vi "UserVars-Plot PDF.vi"(0 "X":dbl[](array[numeric]), 1 "XYGraph":refnum<vi>, 2 "X-axis":refnum<vi>, 5 "PDF":dbl[](array[numeric]), 7 "refpts":dbl[](array[numeric]), 9 "mass":bool, 11 "bernoulli":bool) -> ()   [LabVIEW 2020]
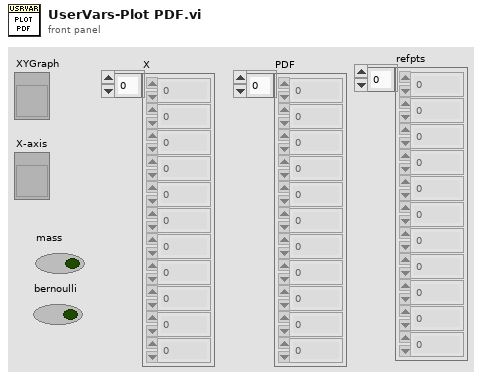
[diagram p1: front panel]
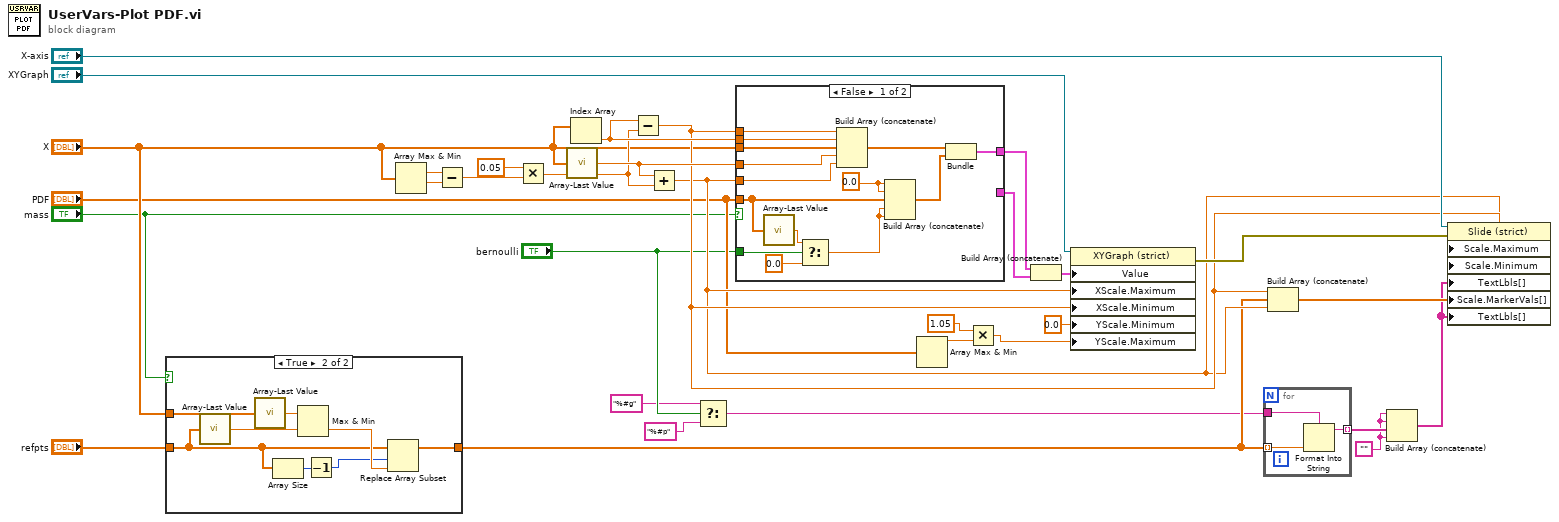
[diagram p0: block diagram]
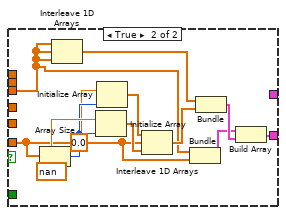
[diagram p3: hidden frame]
diagram:
  w27 = ""
  n1 = case shown="True" "mass" {
    tunnel: "X" -> [_ w41]
    tunnel: [w33 w39] -> w12
    tunnel: "refpts" -> [w33 w37]
    frame False {
    }
    frame True {
      n2 = call "Array-Last Value.vi"("array"=w37) -> ("element"=w40:dbl)
      n3 = call "Array-Last Value.vi"("array"=w41) -> ("element"=w34:dbl)
      n4 = Array Size(array=w37) -> (size(s)=w36:i32)
      n5 = Max & Min(x=w34, y=w40) -> (min(x,y)=w38:dbl)  [unwired: 1 out]
      n6 = Decrement(x=w36) -> (x-1=w35:i32)
      n7 = Replace Array Subset(array=w37, new element=w38, index=w35) -> (w39:dbl[])
    }
  }
  n8 = Array Max & Min(array="X") -> (max value=w25:dbl, min value=w24:dbl)  [unwired: 2 out]
  n9 = Subtract(x=w25, y=w24) -> (x-y=w23:dbl)
  n10 = Multiply(x=0.05, y=w23) -> (x*y=w17:dbl)
  n11 = call "Array-Last Value.vi"("array"="X") -> ("element"=w20:dbl)
  n12 = Index Array(array="X") -> (element=w21:dbl)  [unwired: 1 in]
  n13 = Subtract(x=w21, y=w17) -> (x-y=w19:dbl)
  n14 = Add(x=w20, y=w17) -> (x+y=w18:dbl)
  n15 = Select(t="%#g", s="bernoulli", f="%#p" ("format string")) -> (s? t:f=w2:string)
  n16 = case shown="False" "mass" {
    tunnel: "X" -> [w55 w59]
    tunnel: w21 -> [w54 _]
    tunnel: w20 -> [w53 _]
    tunnel: "PDF" -> [w43 w60]
    tunnel: w19 -> [w52 _]
    tunnel: w18 -> [w51 _]
    tunnel: [w48 _] -> w15
    tunnel: [_ w58] -> w14
    tunnel: "bernoulli" -> [w47 _]
    frame False {
      w44 = 0.0
      n17 = call "Array-Last Value.vi"("array"=w43) -> ("element"=w42:dbl)
      n18 = Select(t=w42, s=w47, f=0.0) -> (s? t:f=w45:dbl)
      n19 = Build Array (concatenate)(w52, w54, w55, w53, w51) -> (w50:dbl[])
      n20 = Build Array (concatenate)(w44, w44, w43, w45, w45) -> (w49:dbl[])
      n21 = Bundle(w50, w49) -> (w48:cluster{dbl[], dbl[]})  [unwired: 1 in]
    }
    frame True {
      n22 = Array Size(array=w60) -> (size(s)=w65:i32)
      n23 = Interleave 1D Arrays(w59, w59, w59) -> (w62:dbl[])
      n24 = Initialize Array(nan ("element"), w65) -> (w66:dbl[])
      n25 = Initialize Array(0.0 ("element"), w65) -> (w63:dbl[])
      n26 = Interleave 1D Arrays(w63, w60, w66) -> (w61:dbl[])
      n27 = Bundle("X"=w59, "PDF"=w60) -> (w56:cluster{"X":dbl[], "PDF":dbl[]})  [unwired: 1 in]
      n28 = Bundle(w62, w61) -> (w57:cluster{dbl[], dbl[]})  [unwired: 1 in]
      n29 = Build Array(w56, w57) -> (w58:cluster{"X":dbl[], "PDF":dbl[]}[])
    }
  }
  n30 = Array Max & Min(array="PDF") -> (max value=w8:dbl)  [unwired: 3 out]
  n31 = Multiply(x=1.05, y=w8) -> (x*y=w7:dbl)
  n32 = Build Array (concatenate)(w15, w14) -> (w16:cluster{"X":dbl[], "PDF":dbl[]}[])
  n33 = property class="XYGraph (strict)"(reference="XYGraph", "Value"=w16, "XScale.Maximum"=w18, "XScale.Minimum"=w19, "YScale.Minimum"=0.0 ("Y Scale.Range:Minimum"), "YScale.Maximum"=w7) -> (error out=w30:errorcluster)  [unwired: 1 in, 1 out]
  n34 = for {
    tunnel: w12 -> [w70] mode=indexing
    tunnel: [w69] -> w28 mode=indexing
    tunnel: w2 -> [w68]
    n35 = Format Into String(format string=w68, w70) -> (resulting string=w69:string)  [unwired: 2 in, 1 out]
  }
  n36 = Build Array (concatenate)(w19, w12, w18) -> (w29:dbl[])
  n37 = Build Array (concatenate)(w27, w27, w28, w27) -> (w26:string[])
  n38 = property class="Slide (strict)"(reference="X-axis", error in=w30, "Scale.Maximum"=w18, "Scale.Minimum"=w19, "TextLbls[]"=w26, "Scale.MarkerVals[]"=w29, "TextLbls[]"=w26) -> ()  [unwired: 2 out]
